vi "LOGinit.vi"(8 "Error In":errorcluster, 11 "LOG file path (user Documents folder)":string) -> (0 "error out":errorcluster)   [LabVIEW 2025, in "LOGlib_LV2025.lvlib"]
uses:
  LOGlib_LV2025.lvlib
  <vilib>/Utility/sysdir.llb/System Directory Type.ctl
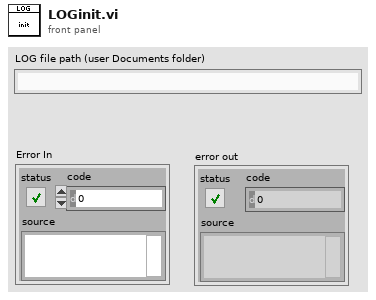
[diagram p1: front panel]
types:
  T1 = typedef "System Directory Type.ctl" = i32
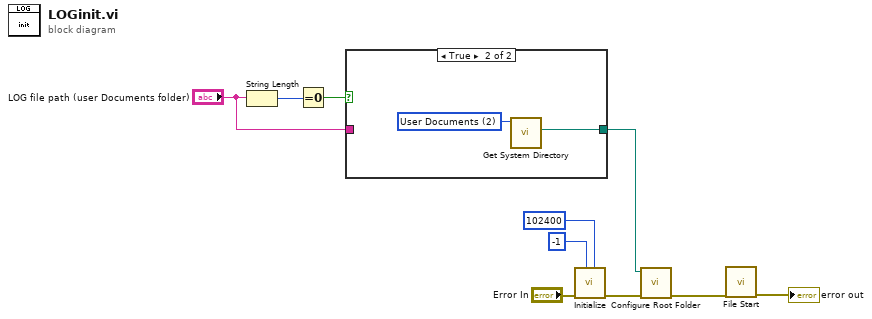
[diagram p0: block diagram]
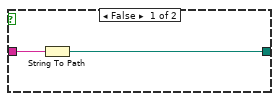
[diagram p2: hidden frame]
diagram:
  n1 = String Length(string="LOG file path (user Documents folder)") -> (length=w5:i32)
  n2 = Equal To 0?(x=w5) -> (x = 0?=w4:bool)
  n3 = case shown="True" w4 {
    tunnel: "LOG file path (user Documents folder)" -> [w12 _]
    tunnel: [w11 w13] -> w2
    frame False {
      n4 = String To Path(string=w12) -> (path=w11:path)
    }
    frame True {
      w14 = T1 2 items=["User Home"=0, "User Desktop"=1, "User Documents"=2, "User Application Data"=3, "User Preferences"=4, "User Temporary"=5, "Public Documents"=6, "Public Application Data"=7, "Public Preferences"=8, "Public Cache"=13, "System Core Libraries"=9, "System Installed Libraries"=10, "Application Files"=11, "Boot Volume Root"=12] ("system directory type")
      n5 = call <vilib>:"Get System Directory.vi"("system directory type"=w14) -> ("system directory"=w13:path)  [unwired: 10 in]
    }
  }
  n6 = call "Initialize.vi"("Buffer Capacity"=102400, "Maximum Messages"=-1, "Error In"="Error In") -> ("Error Out"=w9:errorcluster)  [unwired: 8 in]
  n7 = call "Configure Root Folder.vi"("Error In"=w9, "Root Folder"=w2) -> ("Error Out"=w10:errorcluster)  [unwired: 9 in]
  n8 = call "File Start.vi"("Error In"=w10) -> ("Error Out"=→"error out":errorcluster)  [unwired: 10 in]
